vi "Load.vi"(6 "compatible?":bool, 8 "error in (no error)":errorcluster, 9 "create file if necessary? (T)":bool=TRUE, 10 "configuration file path":path, 11 "queue in":T1) -> (0 "error out":errorcluster, 2 "file created?":bool, 3 "queue out":T1)   [LabVIEW 2020, in "NI_LVConfig.lvlib"]
uses:
  <vilib>/Utility/config.llb/NI_LVConfig.lvlib
  <vilib>/Utility/config.llb/Config Queue.ctl
  <vilib>/Utility/config.llb/Config Data.ctl
  <vilib>/Utility/config.llb/Section.ctl
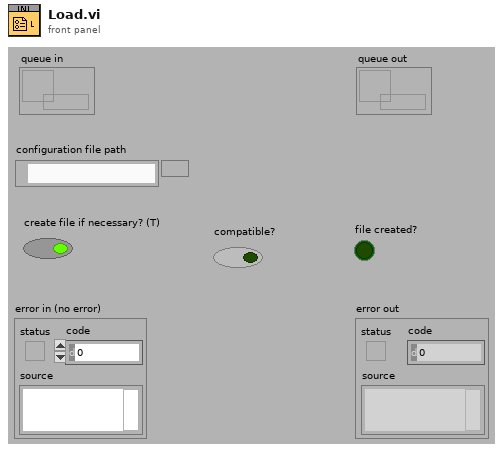
[diagram p1: front panel]
types:
  T1 = typedef "NI_LVConfig.lvlib/Config Queue.ctl" = refnum<queue>
  T2 = typedef "NI_LVConfig.lvlib/Config Data.ctl" = cluster{"sections":T3[], "path":path, "dirty":bool}
  T3 = typedef "NI_LVConfig.lvlib/Section.ctl" = cluster{"name":string, "comment":string, "kvc":string[][]}
  T4 = enum16{"open", "replace", "create", "open or create", "replace or create", "replace or create with confirmation"}
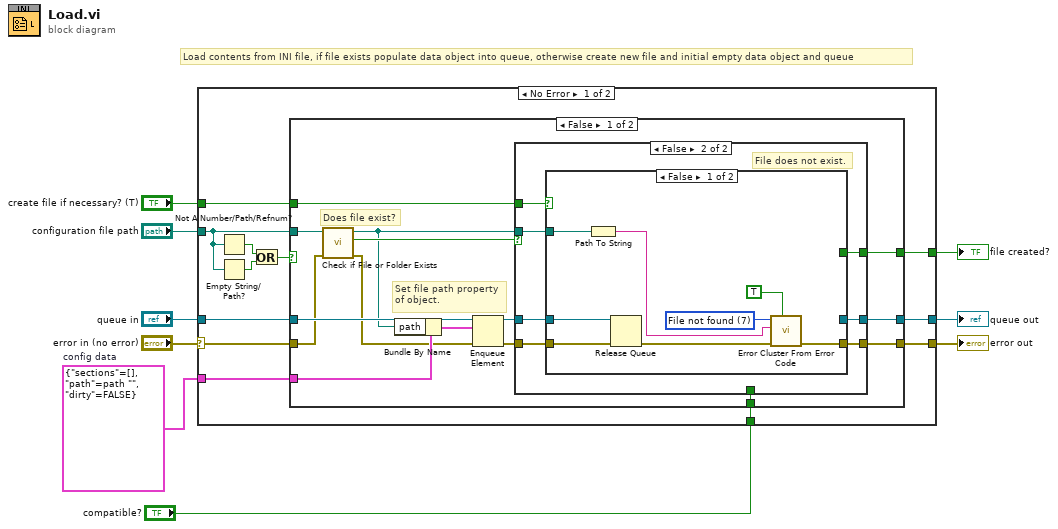
[diagram p0: block diagram]
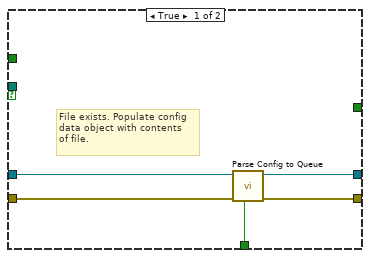
[diagram p2: hidden frame]
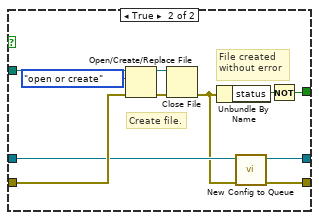
[diagram p3: hidden frame]
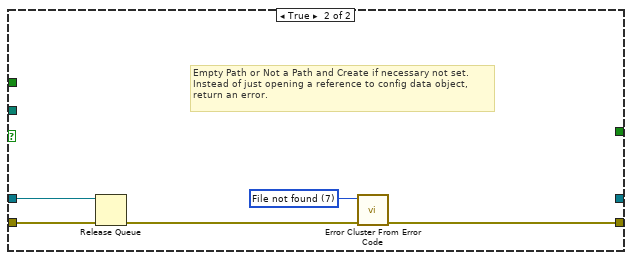
[diagram p4: hidden frame]
diagram:
  w2 = T2 {"sections"=[], "path"=path "", "dirty"=FALSE}  # config data
  # "Load contents from INI file, if file exists populate data object into queue, otherwise create new file and initial empty data object and queue"
  n1 = case shown="No Error" "error in (no error)" {
    selector: "error in (no error)" -> [w17 w74]
    tunnel: [w14 w74] -> w8
    tunnel: [w15 w73] -> w3
    tunnel: "configuration file path" -> [w16 _]
    tunnel: "create file if necessary? (T)" -> [w18 _]
    tunnel: [w13 _] -> w5
    tunnel: "queue in" -> [w12 w73]
    tunnel: w2 -> [w11 _]
    tunnel: "compatible?" -> [w10 _]
    frame No Error {
      n2 = Not A Number/Path/Refnum?(number/path/refnum=w16) -> (NaN/Path/Refnum?=w20:bool)
      n3 = Empty String/Path?(string/path=w16) -> (empty?=w21:bool)
      n4 = Or(x=w20, y=w21) -> (x .or. y?=w19:bool)
      n5 = case shown="False" w19 {
        tunnel: [w36 w72] -> w14
        tunnel: w16 -> [w29 _]
        tunnel: w18 -> [w35 _]
        tunnel: w17 -> [w25 w69]
        tunnel: [w34 _] -> w15
        tunnel: [w33 _] -> w13
        tunnel: w12 -> [w28 w70]
        tunnel: w11 -> [w27 _]
        tunnel: w10 -> [w22 _]
        frame False {
          # "Set file path property\nof object."
          # "Does file exist?"
          n6 = call <vilib>:"Check if File or Folder Exists.vi"("error in (no error)"=w25, "path"=w29) -> ("error out"=w24:errorcluster, "file or folder exists?"=w30:bool, "dup path"=w23:path)  [unwired: 7 out]
          n7 = Bundle By Name(cluster=w27, "path"=w23) -> (w26:T2)
          n8 = Enqueue Element(queue=w28, element=w26, error in (no error)=w24) -> (queue out=w32:T1, error out=w31:errorcluster)  [unwired: 2 out]
          n9 = case shown="False" w30 {
            tunnel: [w40 w47] -> w36
            tunnel: w23 -> [_ w48]
            tunnel: w35 -> [_ w46]
            tunnel: w32 -> [w41 w43]
            tunnel: [w39 w44] -> w34
            tunnel: [_ w45] -> w33
            tunnel: w31 -> [w38 w42]
            tunnel: w22 -> [w37 _]
            frame True {
              # "File exists. Populate config\ndata object with contents\nof file."
              n10 = call <vilib>:"Parse Config to Queue.vi"("compatible?"=w37, "error in"=w38, "queue in"=w41) -> ("error out"=w40:errorcluster, "queue out"=w39:T1)  [unwired: 7 out]
            }
            frame False {
              # "File does not exist."
              n11 = case shown="False" w46 {
                tunnel: w48 -> [w50 w67]
                tunnel: [w55 w60] -> w47
                tunnel: [_ w57] -> w45
                tunnel: [_ w61] -> w44
                tunnel: w43 -> [w54 w62]
                tunnel: w42 -> [w53 w63]
                frame False {
                  w56 = u16 7 items=["No error", "Argument error", "Memory is full", "Out of zone", "End of file", "File already open", "Generic file I/O error", "File not found", "File permission error", "Disk is full", "Duplicate path", "Too many files open", "System feature not enabled", "Resource file not found", "Cannot add resource", "Resource not found", "Image not found", "Image memory error", "Pen does not exist", "Config type invalid", "Config token not found", "Config parse error", "Config memory error", "Bad external code format", "Bad external code offset", "External code not present", "Null window", "Destroy window error", "Null menu", "Print aborted", "Bad print record", "Print driver error", "Windows error during printing", "Memory error during printing", "Print dialog error", "Generic print error", "Invalid device refnum", "Device not found", "Device parameter error", "Device unit error", "Cannot open device", "Device call aborted", "Generic error", "Cancelled by user", "Object ID too low", "Object ID too high", "Object not in heap", "Unknown heap", "Unknown object (invalid DefProc)", "Unknown object (DefProc not in table)", "Message out of range", "Invalid (null) method", "Unknown message", "Manager call not supported", "Bad address", "Network operation in progress", "Network operation timed out", "Connection is busy", "Network attribute not supported", "Network error", "Address in use", "System out of memory", "Connection aborted", "Connection refused", "Not connected", "Already connected", "Connection closed", "Initialization error (interapplication manager)", "Bad occurrence", "Wait on unbound occurrence handler", "Occurrence queue overflow", "Datalog type conflict", "Unused", "Unrecognized type (interapplication manager)", "Memory corrupt", "Failed to make temporary DLL", "Old CIN version", "Drag socket not found", "Failed to load drop-object", "Failed to register OLE object", "Failed to release OLE object", "Format specifier type mismatch", "Unknown format specifier", "Too few format specifiers", "Too many format specifiers", "Scan failed", "Newer CIN version", "OLE Convert", "Runtime menu error", "Password tampered", "Unknown error code"]
                  n12 = Path To String(path=w50) -> (string=w49:string)
                  n13 = Release Queue(queue=w54, error in (no error)=w53) -> (error out=w52:errorcluster)  [unwired: 1 in, 2 out]
                  n14 = call <vilib>:"Error Cluster From Error Code.vi"("show call chain? (False)"=TRUE, "error in (no error)"=w52, "error message (\"\")"=w49, "error code (0)"=w56) -> ("error out"=w55:errorcluster)  [unwired: 5 out]
                }
                frame True {
                  # "File created\nwithout error"
                  # "Create file."
                  n15 = Open/Create/Replace File(file path (use dialog)=w67, error in=w63, operation (0:open)=T4."open or create") -> (refnum out=w65:refnum<file>, error out=w66:errorcluster)  [unwired: 4 out]
                  n16 = Close File(refnum=w65, error in=w66) -> (error out=w58:errorcluster)  [unwired: 1 out]
                  n17 = Unbundle By Name(w58) -> ("status"=w59:bool)
                  n18 = call <vilib>:"New Config to Queue.vi"("error in"=w58, "queue in"=w62) -> ("error out"=w60:errorcluster, "queue out"=w61:T1)  [unwired: 8 out]
                  n19 = Not(x=w59) -> (.not. x?=w57:bool)
                }
              }
            }
          }
        }
        frame True {
          w71 = u16 7 items=["No error", "Argument error", "Memory is full", "Out of zone", "End of file", "File already open", "Generic file I/O error", "File not found", "File permission error", "Disk is full", "Duplicate path", "Too many files open", "System feature not enabled", "Resource file not found", "Cannot add resource", "Resource not found", "Image not found", "Image memory error", "Pen does not exist", "Config type invalid", "Config token not found", "Config parse error", "Config memory error", "Bad external code format", "Bad external code offset", "External code not present", "Null window", "Destroy window error", "Null menu", "Print aborted", "Bad print record", "Print driver error", "Windows error during printing", "Memory error during printing", "Print dialog error", "Generic print error", "Invalid device refnum", "Device not found", "Device parameter error", "Device unit error", "Cannot open device", "Device call aborted", "Generic error", "Cancelled by user", "Object ID too low", "Object ID too high", "Object not in heap", "Unknown heap", "Unknown object (invalid DefProc)", "Unknown object (DefProc not in table)", "Message out of range", "Invalid (null) method", "Unknown message", "Manager call not supported", "Bad address", "Network operation in progress", "Network operation timed out", "Connection is busy", "Network attribute not supported", "Network error", "Address in use", "System out of memory", "Connection aborted", "Connection refused", "Not connected", "Already connected", "Connection closed", "Initialization error (interapplication manager)", "Bad occurrence", "Wait on unbound occurrence handler", "Occurrence queue overflow", "Datalog type conflict", "Unused", "Unrecognized type (interapplication manager)", "Memory corrupt", "Failed to make temporary DLL", "Old CIN version", "Drag socket not found", "Failed to load drop-object", "Failed to register OLE object", "Failed to release OLE object", "Format specifier type mismatch", "Unknown format specifier", "Too few format specifiers", "Too many format specifiers", "Scan failed", "Newer CIN version", "OLE Convert", "Runtime menu error", "Password tampered", "Unknown error code"]
          # "Empty Path or Not a Path and Create if necessary not set.\nInstead of just opening a reference to config data object,\nreturn an error."
          n20 = Release Queue(queue=w70, error in (no error)=w69) -> (error out=w68:errorcluster)  [unwired: 1 in, 2 out]
          n21 = call <vilib>:"Error Cluster From Error Code.vi"("error in (no error)"=w68, "error code (0)"=w71) -> ("error out"=w72:errorcluster)  [unwired: 1 in, 6 out]
        }
      }
    }
    frame Error {
    }
  }
  "error out" <- w8
  "file created?" <- w5
  "queue out" <- w3
